vi "SP Format Markers Array for Storage.vi"(7 "Marker Values (none)":dbl[](array[numeric])) -> (3 "Marker":dbl[](array[numeric]))   [LabVIEW 2011]
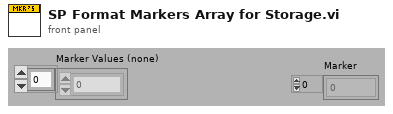
[diagram p1: front panel]
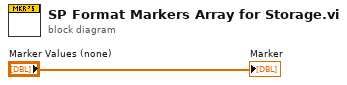
[diagram p0: block diagram]
diagram:
  "Marker" <- "Marker Values (none)"
